vi "Test method finding benchmark.vi"() -> ()   [LabVIEW 2020]
uses:
  tests/Test Doubles/Test Case Test Double/Test Case Test Double.lvclass
  <vilib>/xml/Load XML File.vi
  <vilib>/xml/Close Reference(Node).vi
  <vilib>/xml/NI_XML.lvlib
  <resource>/objmgr/DOMUserDefRef.rc
  <vilib>/xml/Close Reference(NNMap).vi
panel:
  out "Array":path[](array[path])
  out "Array 7":path[](array[path])
  out "Numeric":i32
  out "Array 6":path[](array[path])
  out "appended array":path[](array[path])
  out "Array 2":path[](array[path])
  out "Array 5":path[](array[path])
  out "Array 4":string[](array[string])
  out "Array 3":path[](array[path])
  out "x-y":u32
  # "Name=\"_Test Dynamic Method.vi\" Type=\"VI\" URL=\"../_Test Dynamic Method.vi\">\n\t\t<Property Name=\"NI.ClassItem.ConnectorPane\" Type=\"Bin\">)!#!!!!!!!)!\"1!&amp;!!!-!%!!!@````]!!!!\"!!%!!!&amp;\"!!!!#1!-1#%'=X2B&gt;(6T!!!,1!-!\"'.P:'5!!\"\"!-0````]'=W^V=G.F!!!71&amp;!!!Q!!!!%!!AFF=H*P=C\"P&gt;81!\"!!!!%*!=!!?!!!@(62F=X1A1W&amp;T:3\"5:8.U)%2P&gt;7*M:3ZM&gt;G.M98.T!\"F5:8.U)%.B=W5A6'6T&gt;#\"%&lt;X6C&lt;'5A&lt;X6U!#\"!5!!$!!!!!1!#%W6S=G^S)'FO)#BO&lt;S\"F=H*P=CE!1E\"Q!\"Y!!\"]&gt;6'6T&gt;#\"$98.F)&amp;2F=X1A2'^V9GRF,GRW9WRB=X-!'&amp;2F=X1A1W&amp;T:3\"5:8.U)%2P&gt;7*M:3\"J&lt;A!!6!$Q!!Q!!Q!%!!1!\"1!%!!1!\"!!%!!9!\"!!%!!=$!!\"Y!!!.#!!!!!!!!!!!!!#.#Q!!!!!!!!!!!!!!!!!!!!!!!!I!!!!!!!!!!!!!!*)!!!!!!1!)!!!!!!</Property>\n\t\t<Property Name=\"NI.ClassItem.ExecutionSystem\" Type=\"Int\">-1</Property>\n\t\t<Property Name=\"NI.ClassItem.Flags\" Type=\"Int\">128</Property>\n\t\t<Property Name=\"NI.ClassItem.IsStaticMethod\" Type=\"Bool\">false</Property>\n\t\t<Property Name=\"NI.ClassItem.MethodScope\" Type=\"UInt\">1</Property>\n\t\t<Property Name=\"NI.ClassItem.Priority\" Type=\"Int\">1</Property>\n\t\t<Property Name=\"NI.ClassItem.State\" Type=\"Int\">1074541072</Property>"
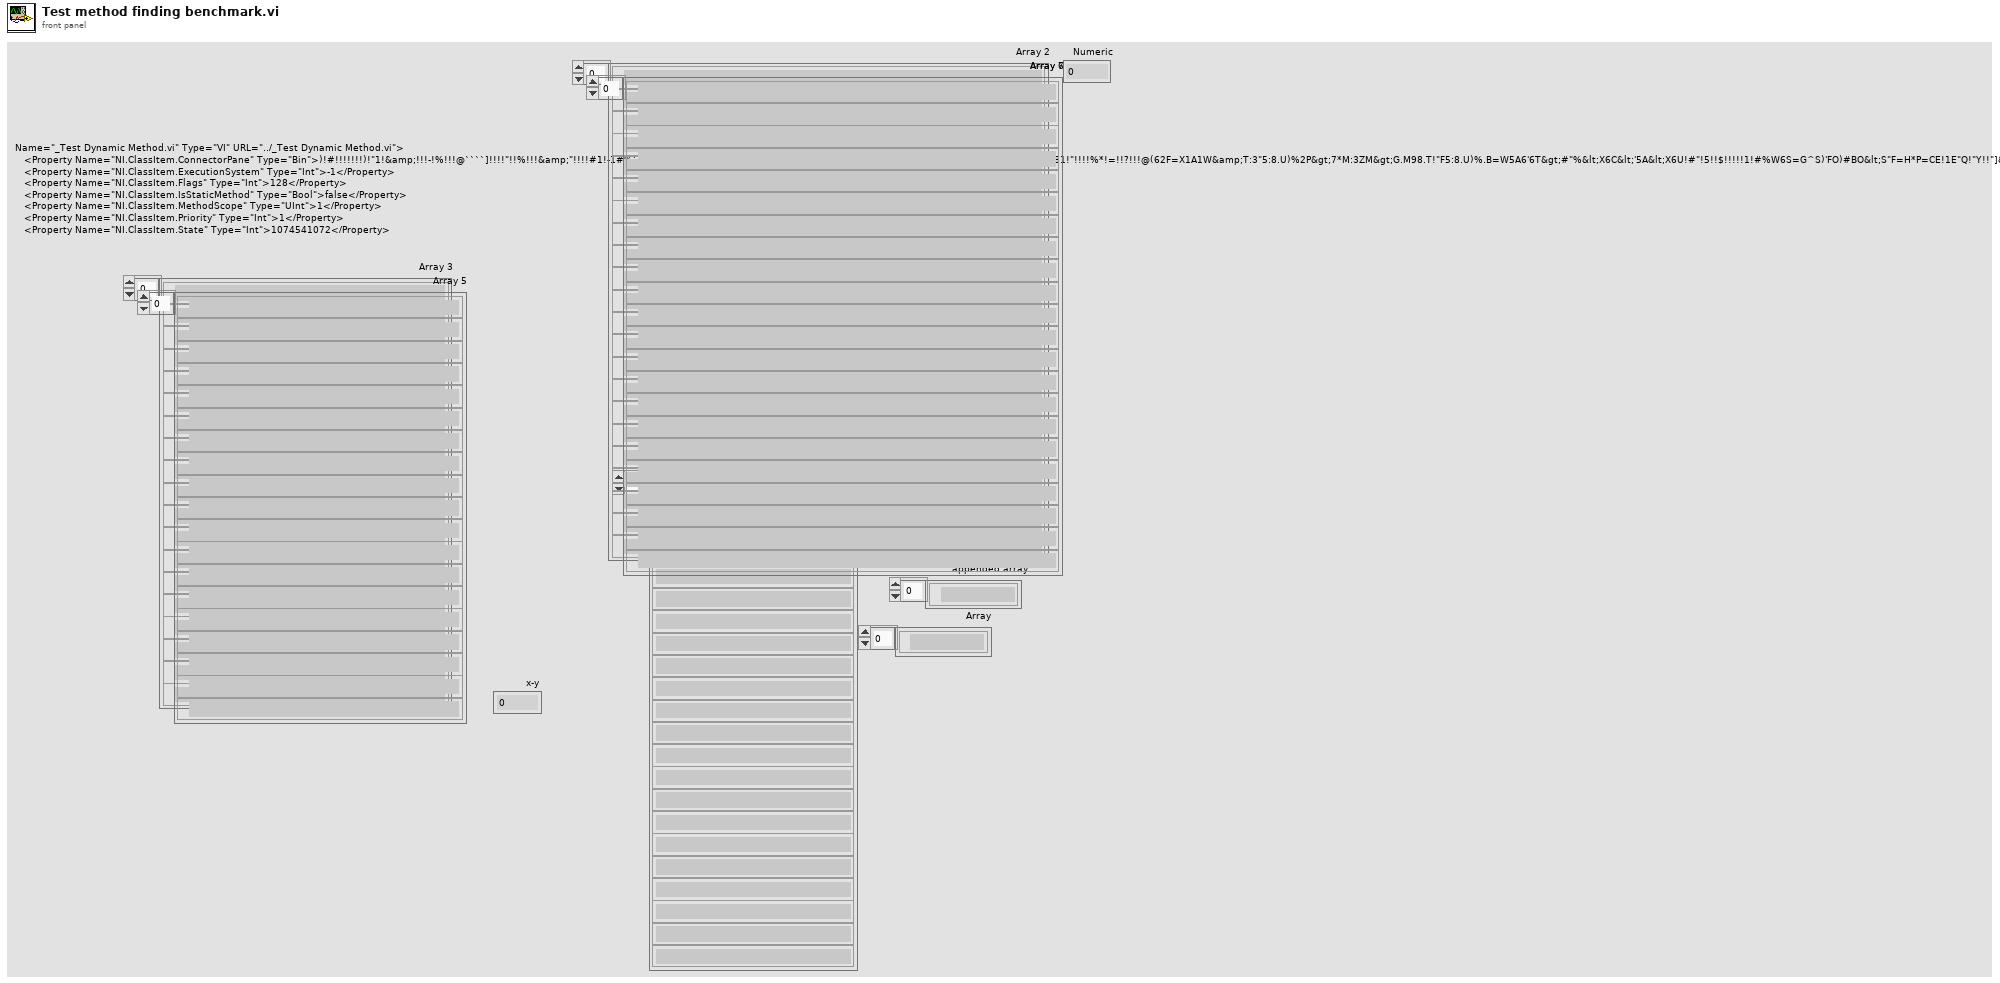
[diagram p1: front panel]
types:
  T1 = enum32{"invalid scope", "public", "private", "protected", "community"}
  T2 = enum16{"open", "replace", "create", "open or create", "replace or create", "replace or create with confirmation"}
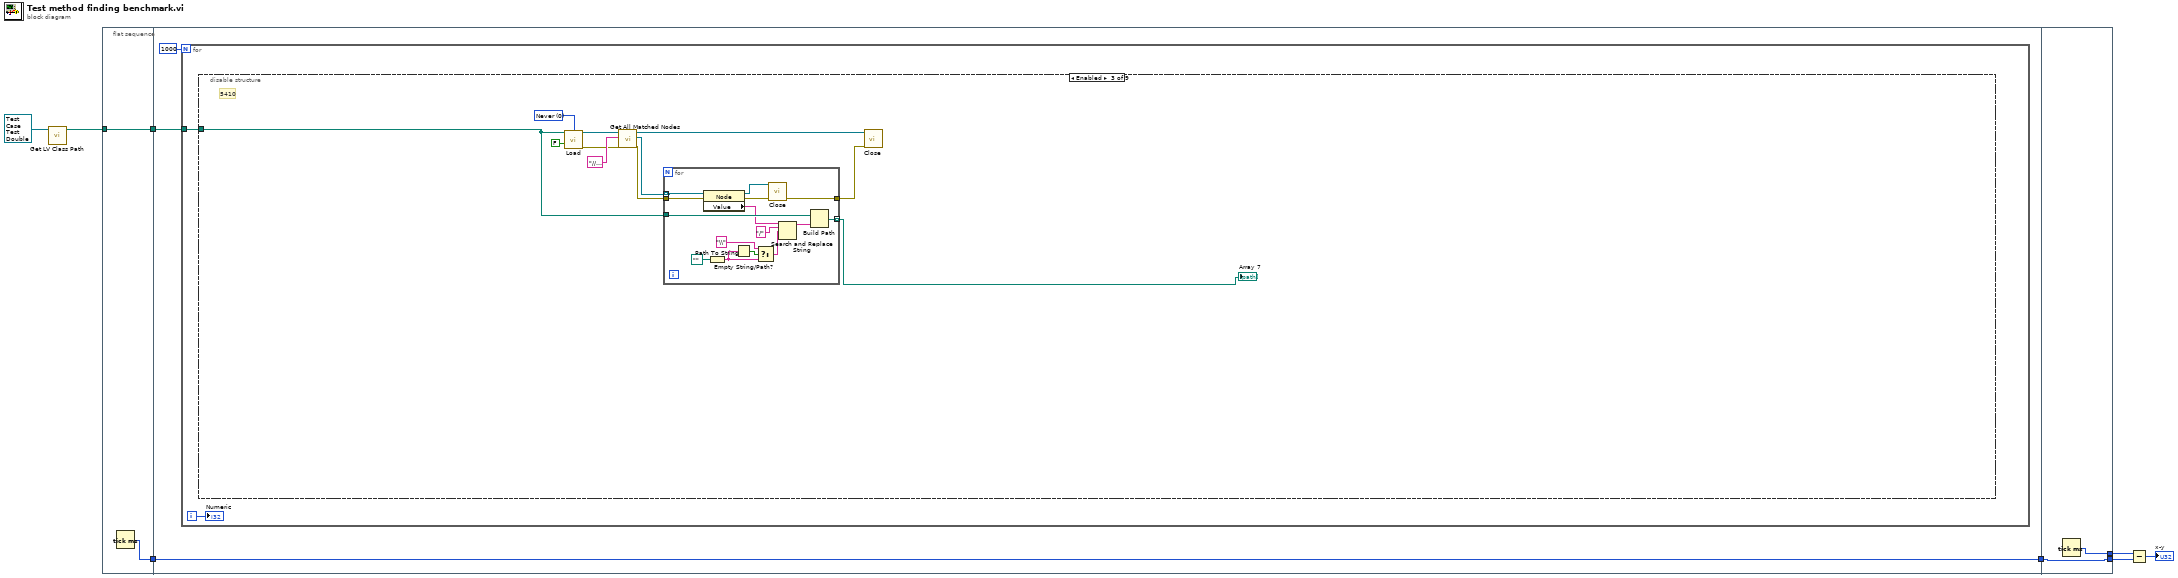
[diagram p0: block diagram]
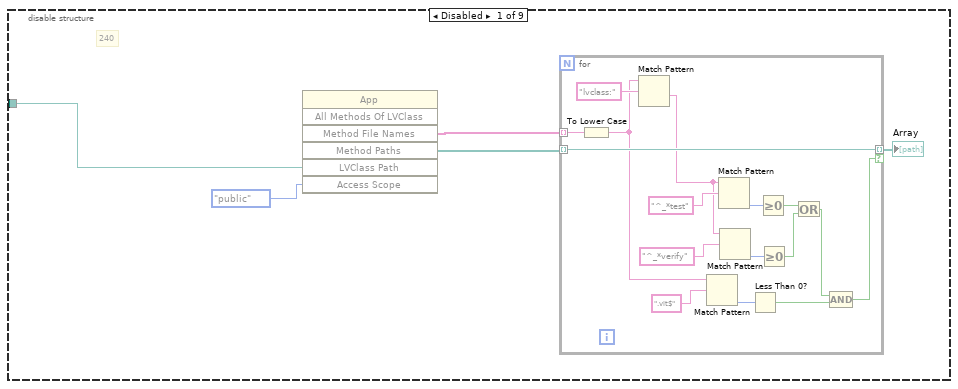
[diagram p2: hidden frame]
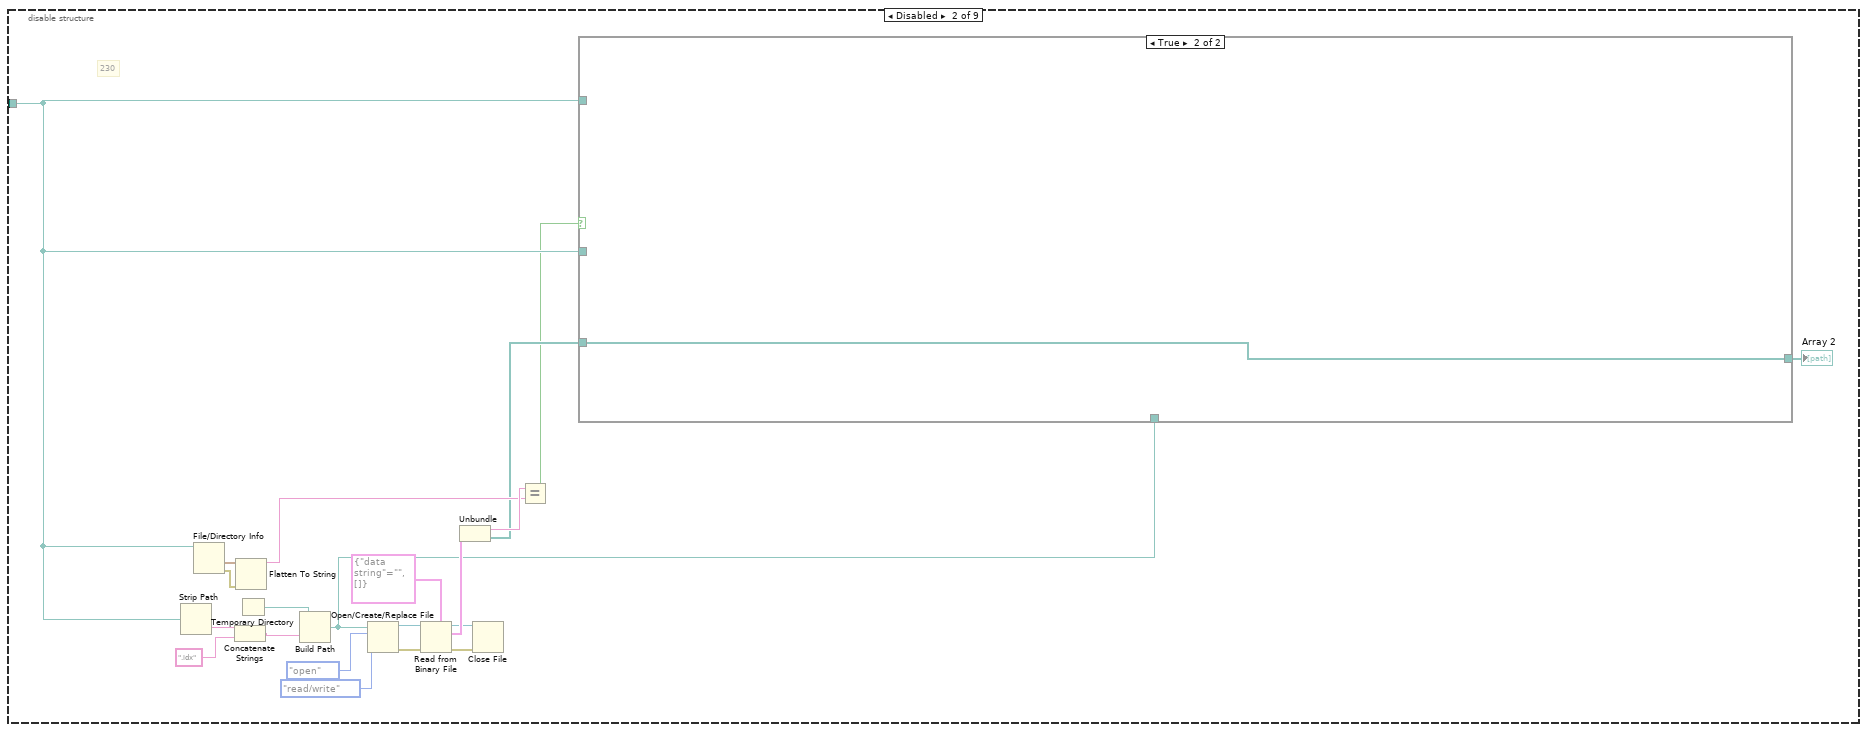
[diagram p3: hidden frame]
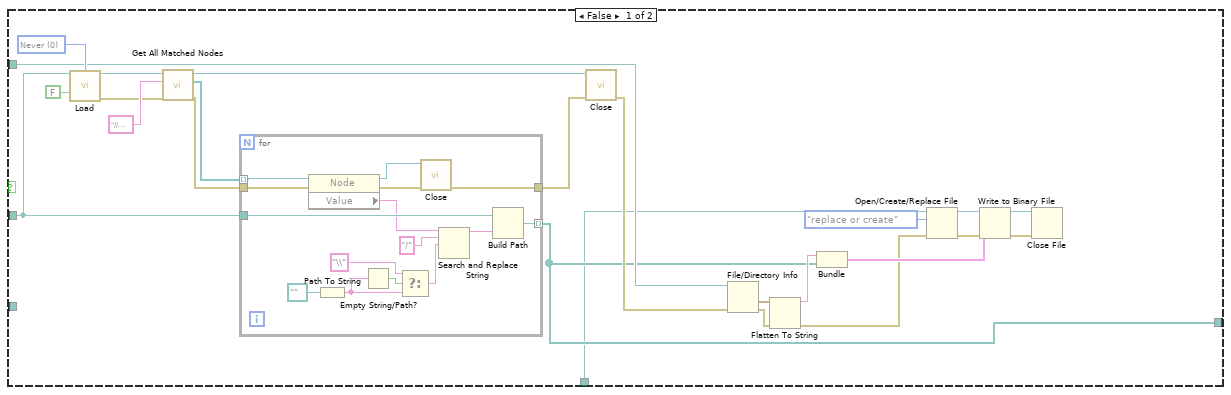
[diagram p4: hidden frame]
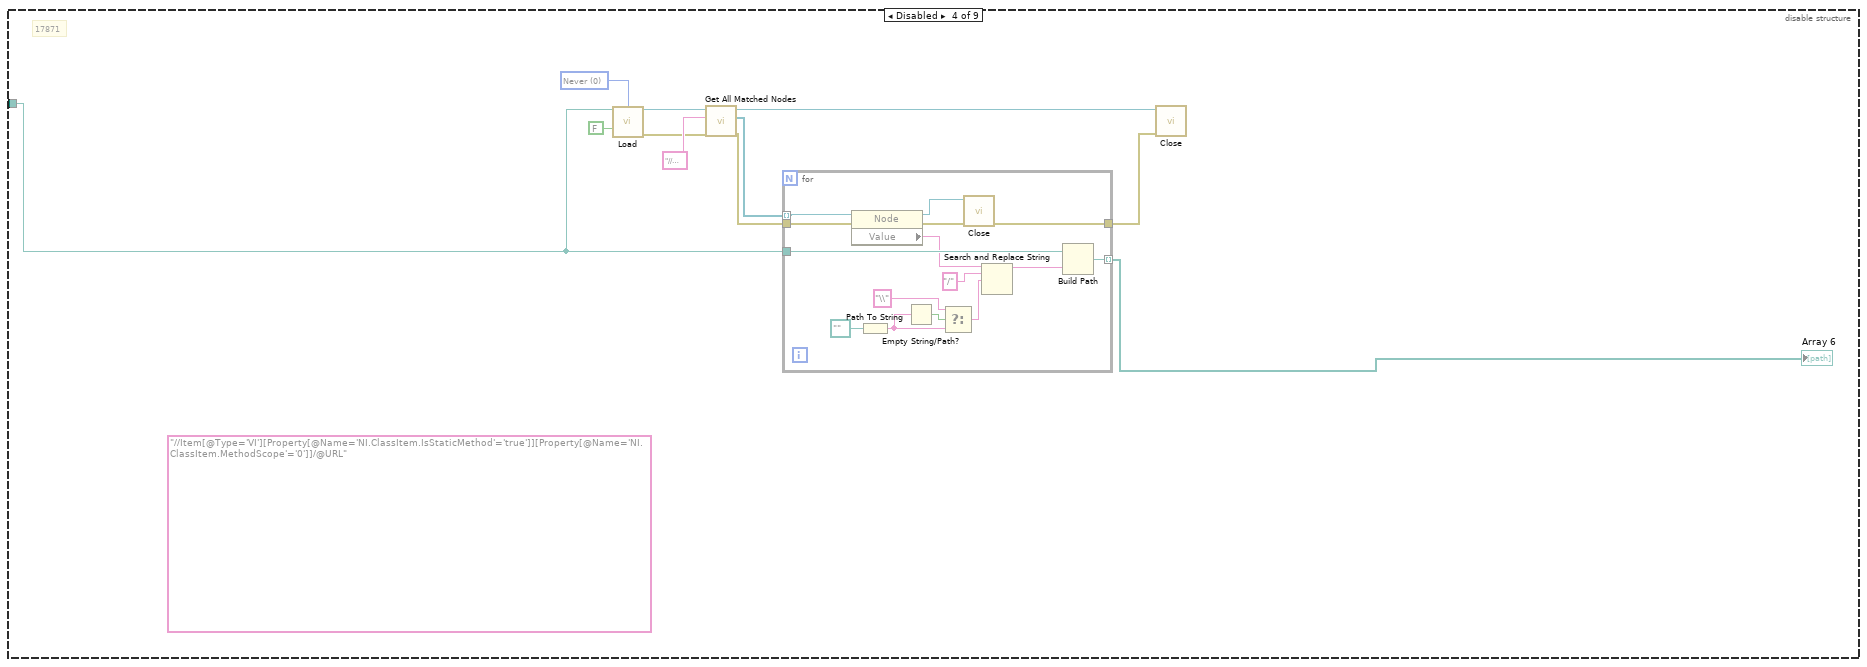
[diagram p5: hidden frame]
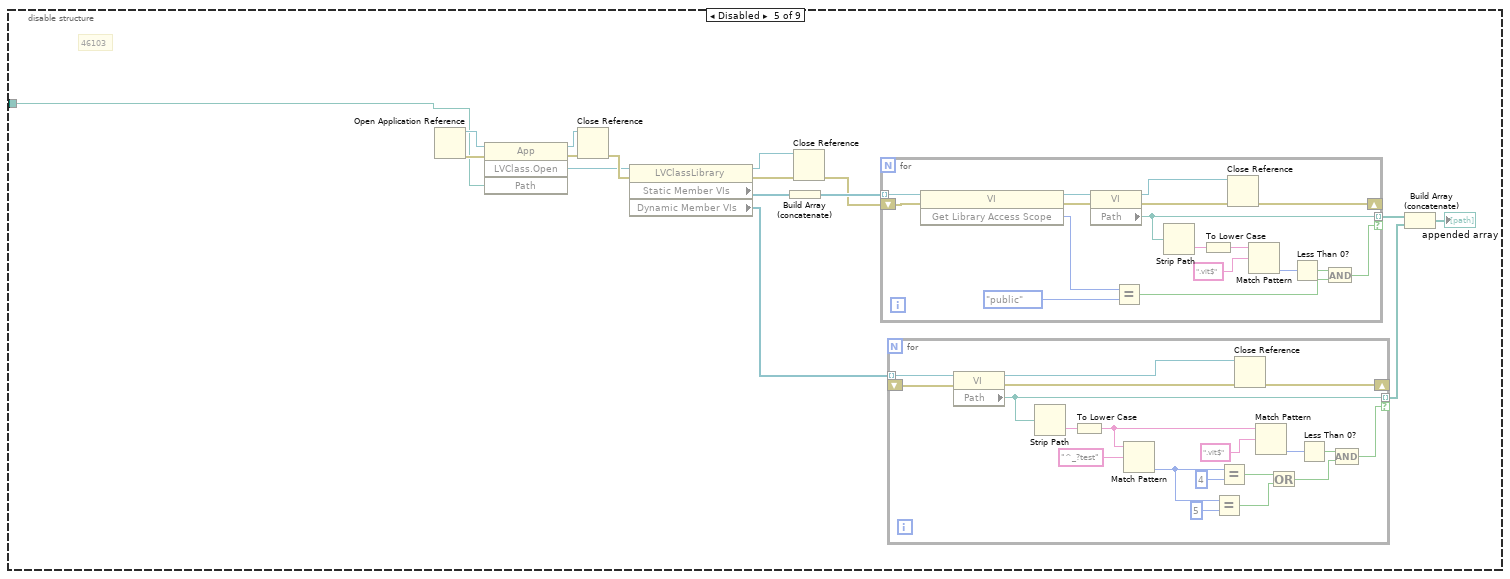
[diagram p6: hidden frame]
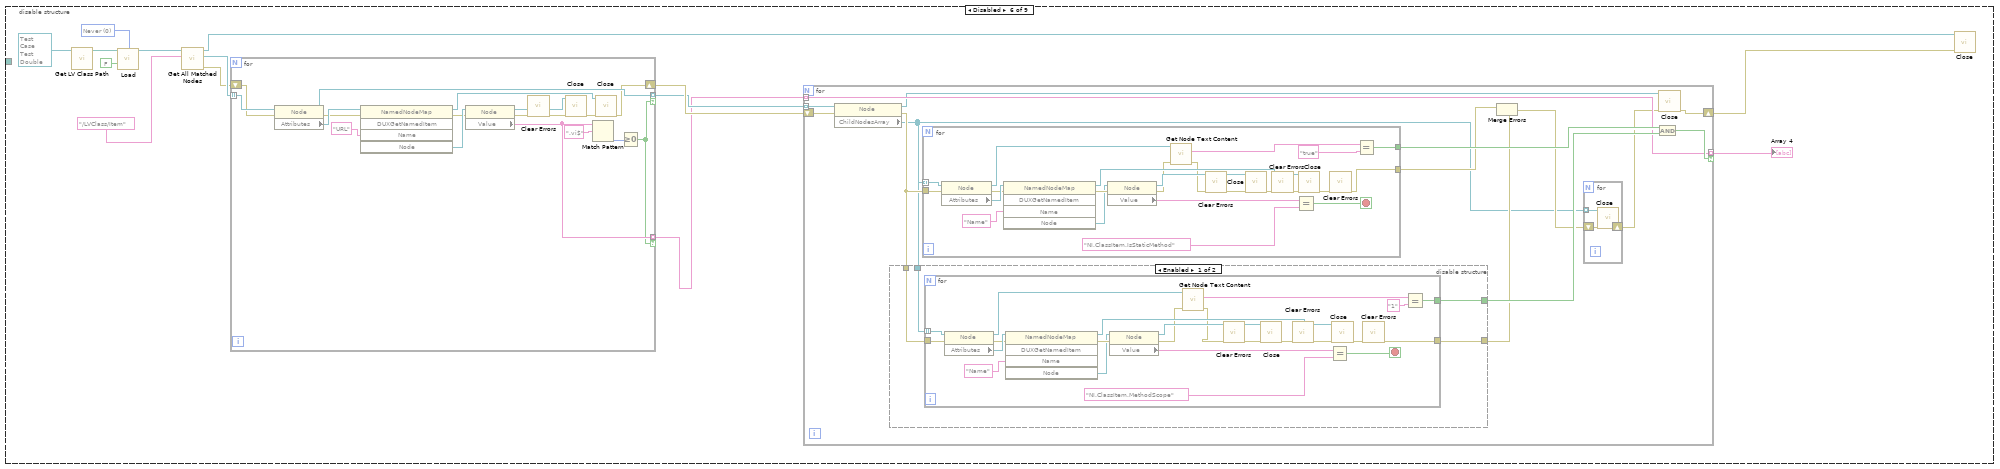
[diagram p7: hidden frame]
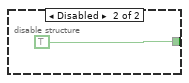
[diagram p8: hidden frame]
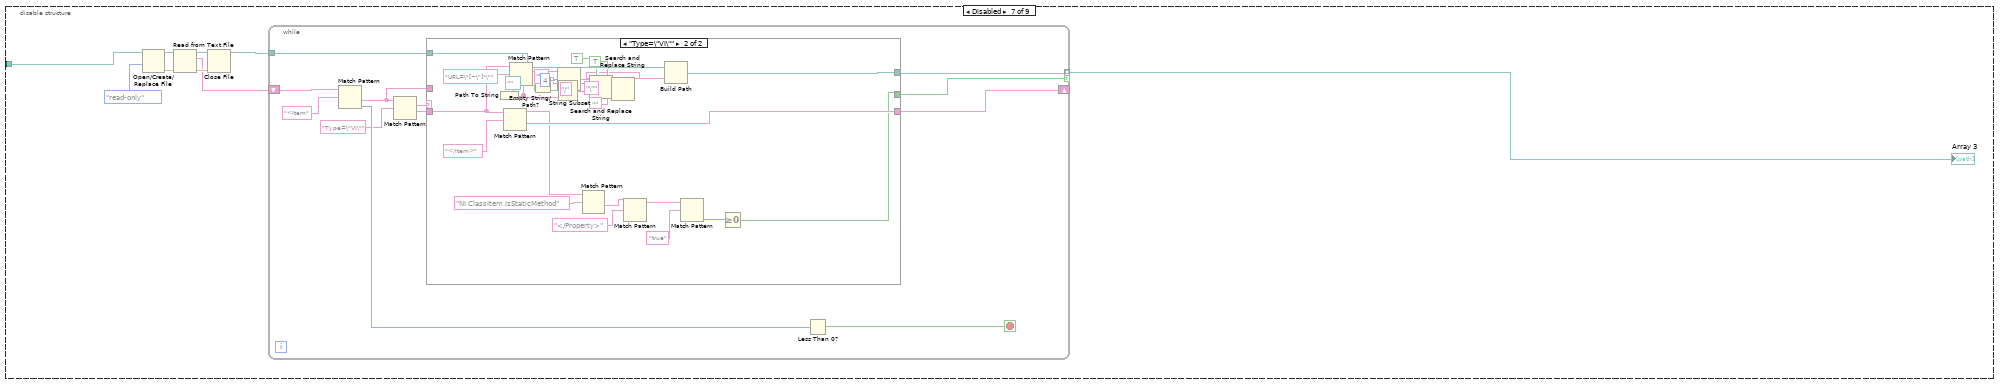
[diagram p9: hidden frame]
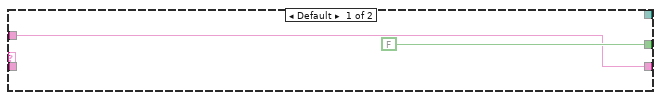
[diagram p10: hidden frame]
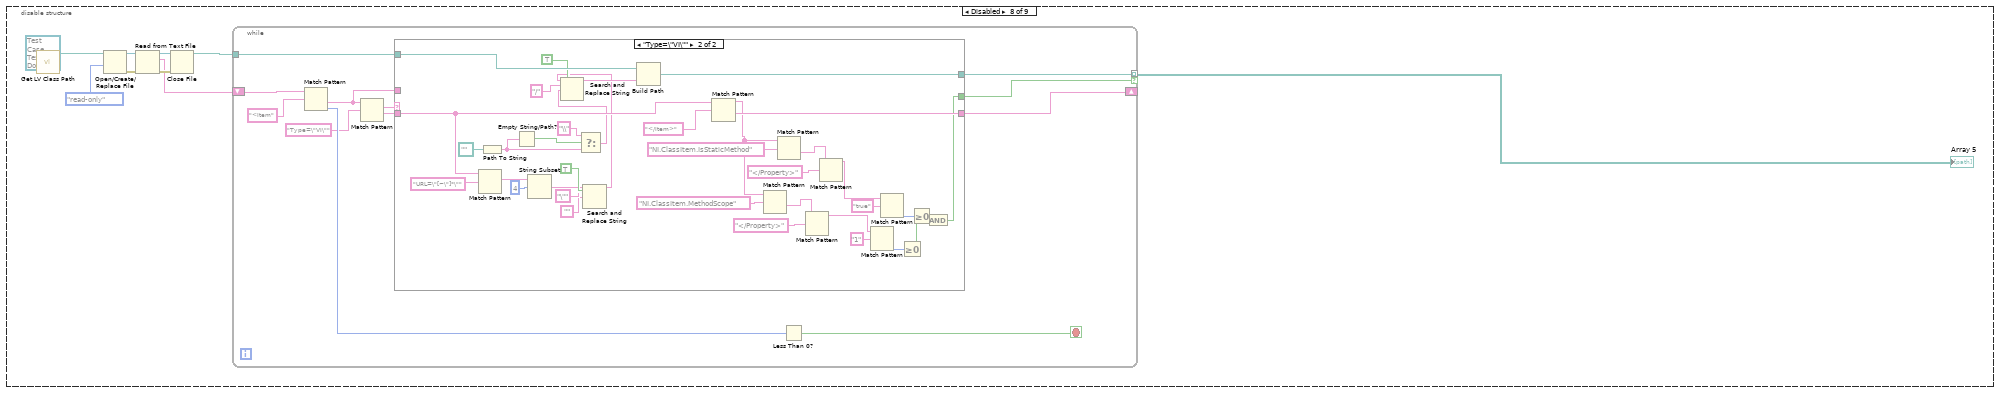
[diagram p11: hidden frame]
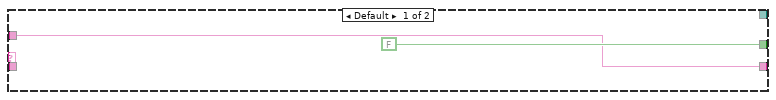
[diagram p12: hidden frame]
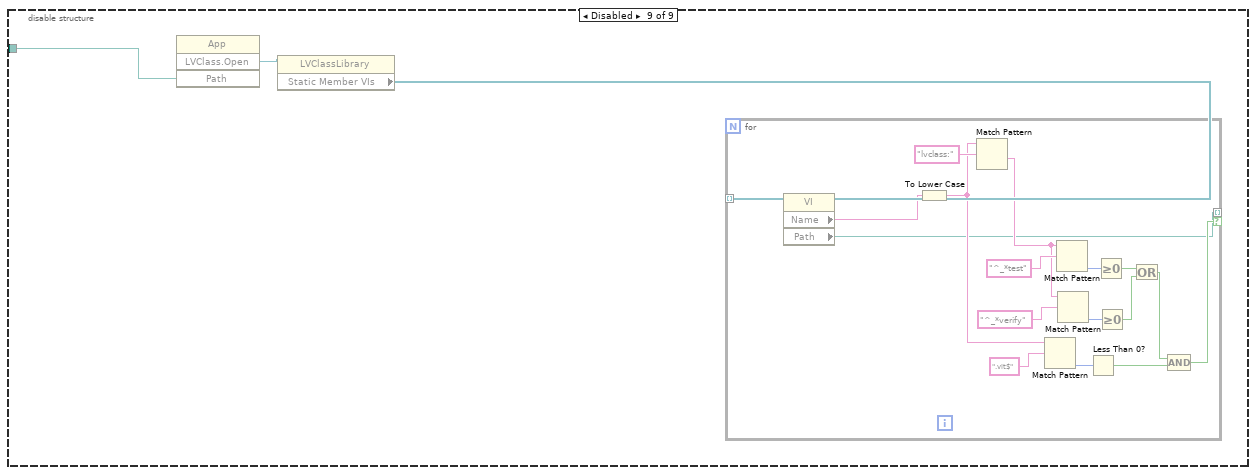
[diagram p13: hidden frame]
diagram:
  n1 = call <vilib>:"Get LV Class Path.vi"("object"=refnum<class "Test Case Test Double.lvclass"> refnum ("Test Case Test Double.lvclass")) -> ("class path"=w2:path)  [unwired: 9 in, 1 out]
  n2 = flat-sequence {
    tunnel: [w10] -> w7
    tunnel: [w9] -> w3
    tunnel: w2 -> [w9]
    tunnel: w7 -> [w13]
    tunnel: [w13] -> w6
    tunnel: w3 -> [w11]
    tunnel: [w437] -> w8
    tunnel: w6 -> [w436]
    tunnel: [w436] -> w5
    frame #0 {
      n3 = Tick Count (ms)() -> (millisecond timer value=w10:u32)
    }
    frame #1 {
      n4 = for {
        N: 1000 -> [_]
        tunnel: w11 -> [w15]
        i -> [w14]
        n5 = disable-structure shown="Enabled" {
          disable-tunnel: w15 -> [w16 w45 w107 w133 w151 _ w302 _ w415]
          frame Disabled {
            # "240"
            n6 = invoke class="App" method="All Methods Of LVClass"("LVClass Path"=w16, "Access Scope"=T1."public") -> ("Method File Names"=w18:string[], "Method Paths"=w19:path[])  [unwired: 5 in, 5 out]
            n7 = for {
              tunnel: [w32] -> w17 mode=indexing if=w33
              tunnel: w19 -> [w32] mode=indexing
              tunnel: w18 -> [w28] mode=indexing
              n8 = To Lower Case(string=w28) -> (all lower case string=w22:string)
              n9 = Match Pattern(string=w22, regular expression="lvclass:") -> (after substring=w29:string)  [unwired: 1 in, 3 out]
              n10 = Match Pattern(string=w22, regular expression=".vit$") -> (offset past match=w35:i32)  [unwired: 1 in, 3 out]
              n11 = Match Pattern(string=w29, regular expression="^_*test") -> (offset past match=w31:i32)  [unwired: 1 in, 3 out]
              n12 = Match Pattern(string=w29, regular expression="^_*verify") -> (offset past match=w25:i32)  [unwired: 1 in, 3 out]
              n13 = Less Than 0?(x=w35) -> (x < 0?=w34:bool)
              n14 = Greater Or Equal To 0?(x=w31) -> (x >= 0?=w23:bool)
              n15 = Greater Or Equal To 0?(x=w25) -> (x >= 0?=w24:bool)
              n16 = Or(x=w23, y=w24) -> (x .or. y?=w21:bool)
              n17 = Compound Arithmetic op=AND(w21, w34) -> (w33:bool)
            }
            "Array" <- w17
          }
          frame Disabled {
            # "230"
            n18 = Strip Path(path=w45) -> (name=w57:string)  [unwired: 1 out]
            n19 = File/Directory Info(path=w45) -> (last mod=w43:timestamp, error out=w44:errorcluster)  [unwired: 1 in, 5 out]
            n20 = Concatenate Strings(w57, ".idx" ("string")) -> (w54:string)
            n21 = Flatten To String(anything=w43, error in (no error)=w44) -> (data string=w49:string)  [unwired: 2 in, 2 out]
            n22 = Temporary Directory() -> (w55:path)
            n23 = Build Path(base path=w55, name or relative path=w54) -> (appended path=w47:path)
            n24 = Open/Create/Replace File(file path (use dialog)=w47, operation (0:open)=T2."open", access (0:read/write)=enum16{"read/write", "read-only", "write-only"}."read/write") -> (refnum out=w42:refnum<file>, error out=w41:errorcluster)  [unwired: 3 in, 1 out]
            n25 = Read from Binary File(5:cluster{"data string":string, path[]} {"data string"="", []} ("output cluster"), 8:w41, 11:w42) -> (0:w39:errorcluster, 2:w51:cluster{"data string":string, path[]}, 3:w40:refnum<file>)  [unwired: 3 in, 1 out]
            n26 = Unbundle(w51) -> ("data string"=w50:string, w48:path[])
            n27 = Close File(refnum=w40, error in=w39) -> ()  [unwired: 2 out]
            n28 = Equal?(x=w50, y=w49) -> (x = y?=w37:bool)
            n29 = case shown="True" w37 {
              tunnel: [w66 w97] -> w46
              tunnel: w45 -> [w72 _]
              tunnel: w48 -> [_ w97]
              tunnel: w45 -> [w68 _]
              tunnel: w47 -> [w61 _]
              frame False {
                w81 = 0 items=["Never", "Always", "Auto"] ("validate on load (Auto)")
                n30 = call-poly <vilib>:"Load.vi"("path to XML document"=w72, "validate on load (Auto)"=w81, "load external DTD (True)"=FALSE) -> ("DOM document out"=w79:refnum<k20>, "error out"=w73:errorcluster)  [unwired: 10 in, 1 out]
                n31 = call <vilib>:"Get All Matched Nodes.vi"("error in (no error)"=w73, "XPath expression"="//Item[@Type='VI'][Property[@Name='NI.ClassItem.IsStaticMethod'='true']][Property[@Name='NI.ClassItem.MethodScope'='0']]/@URL", "node in"=w79) -> ("error out"=w75:errorcluster, "node result array"=w77:refnum<k20>[], "node out"=w76:refnum<k20>)  [unwired: 6 out]
                n32 = for {
                  tunnel: w77 -> [w96] mode=indexing
                  tunnel: w75 -> [w95]
                  tunnel: [w92] -> w74
                  tunnel: w72 -> [w84]
                  tunnel: [w83] -> w66 mode=indexing
                  n33 = property class="Node"(reference=w96, error in=w95) -> (reference out=w94:refnum<k20>, error out=w93:errorcluster, "Value"=w82:string)
                  n34 = Path To String(path=path "") -> (string=w90:string)
                  n35 = Empty String/Path?(string/path=w90) -> (empty?=w89:bool)
                  n36 = Select(t="\\" ("search string"), s=w89, f=w90) -> (s? t:f=w88:string)
                  n37 = call-poly <vilib>:"Close.vi"("error in (no error)"=w93, "node"=w94) -> ("error out"=w92:errorcluster)  [unwired: 7 out]
                  n38 = Search and Replace String(input string=w82, search string="/", replace string=w88) -> (result string=w91:string)  [unwired: 5 in, 3 out]
                  n39 = Build Path(base path=w84, name or relative path=w91) -> (appended path=w83:path)
                }
                n40 = call-poly <vilib>:"Close.vi"("error in (no error)"=w74, "node"=w76) -> ("error out"=w69:errorcluster)  [unwired: 7 out]
                n41 = File/Directory Info(path=w68, error in=w69) -> (last mod=w70:timestamp, error out=w71:errorcluster)  [unwired: 5 out]
                n42 = Flatten To String(anything=w70, error in (no error)=w71) -> (data string=w67:string, error out=w58:errorcluster)  [unwired: 2 in, 1 out]
                n43 = Bundle("data string"=w67, w66) -> (w60:cluster{"data string":string, path[]})  [unwired: 1 in]
                n44 = Open/Create/Replace File(file path (use dialog)=w61, error in=w58, operation (0:open)=T2."replace or create") -> (refnum out=w62:refnum<file>, error out=w63:errorcluster)  [unwired: 3 in, 1 out]
                n45 = Write to Binary File(file (use dialog)=w62, data=w60, error in=w63) -> (refnum out=w64:refnum<file>, error out=w65:errorcluster)  [unwired: 3 in, 1 out]
                n46 = Close File(refnum=w64, error in=w65) -> ()  [unwired: 2 out]
              }
              frame True {
              }
            }
            "Array 2" <- w46
          }
          frame Enabled {
            w106 = 0 items=["Never", "Always", "Auto"] ("validate on load (Auto)")
            # "5410"
            n47 = call-poly <vilib>:"Load.vi"("path to XML document"=w107, "validate on load (Auto)"=w106, "load external DTD (True)"=FALSE) -> ("DOM document out"=w104:refnum<k20>, "error out"=w98:errorcluster)  [unwired: 10 in, 1 out]
            n48 = call <vilib>:"Get All Matched Nodes.vi"("error in (no error)"=w98, "XPath expression"="//Item[@Type='VI'][Property[@Name='NI.ClassItem.IsStaticMethod'='true']][Property[@Name='NI.ClassItem.MethodScope'='0']]/@URL", "node in"=w104) -> ("error out"=w100:errorcluster, "node result array"=w102:refnum<k20>[], "node out"=w101:refnum<k20>)  [unwired: 6 out]
            n49 = for {
              tunnel: w102 -> [w123] mode=indexing
              tunnel: w100 -> [w122]
              tunnel: [w119] -> w99
              tunnel: w107 -> [w111]
              tunnel: [w110] -> w108 mode=indexing
              n50 = property class="Node"(reference=w123, error in=w122) -> (reference out=w121:refnum<k20>, error out=w120:errorcluster, "Value"=w109:string)
              n51 = Path To String(path=path "") -> (string=w117:string)
              n52 = Empty String/Path?(string/path=w117) -> (empty?=w116:bool)
              n53 = Select(t="\\" ("search string"), s=w116, f=w117) -> (s? t:f=w115:string)
              n54 = call-poly <vilib>:"Close.vi"("error in (no error)"=w120, "node"=w121) -> ("error out"=w119:errorcluster)  [unwired: 7 out]
              n55 = Search and Replace String(input string=w109, search string="/", replace string=w115) -> (result string=w118:string)  [unwired: 5 in, 3 out]
              n56 = Build Path(base path=w111, name or relative path=w118) -> (appended path=w110:path)
            }
            "Array 7" <- w108
            n57 = call-poly <vilib>:"Close.vi"("error in (no error)"=w99, "node"=w101) -> ()  [unwired: 8 out]
          }
          frame Disabled {
            (unwired) "//Item[@Type='VI'][Property[@Name='NI.ClassItem.IsStaticMethod'='true']][Property[@Name='NI.ClassItem.MethodScope'='0']]/@URL" ("XPath expression")
            w132 = 0 items=["Never", "Always", "Auto"] ("validate on load (Auto)")
            # "17871"
            n58 = call-poly <vilib>:"Load.vi"("path to XML document"=w133, "validate on load (Auto)"=w132, "load external DTD (True)"=FALSE) -> ("DOM document out"=w130:refnum<k20>, "error out"=w124:errorcluster)  [unwired: 10 in, 1 out]
            n59 = call <vilib>:"Get All Matched Nodes.vi"("error in (no error)"=w124, "XPath expression"="//Item[@Type='VI'][Property[@Name='NI.ClassItem.IsStaticMethod']='true'][Property[@Name='NI.ClassItem.MethodScope']='1']/@URL", "node in"=w130) -> ("error out"=w126:errorcluster, "node result array"=w128:refnum<k20>[], "node out"=w127:refnum<k20>)  [unwired: 6 out]
            n60 = for {
              tunnel: w128 -> [w149] mode=indexing
              tunnel: w126 -> [w148]
              tunnel: [w145] -> w125
              tunnel: w133 -> [w137]
              tunnel: [w136] -> w134 mode=indexing
              n61 = property class="Node"(reference=w149, error in=w148) -> (reference out=w147:refnum<k20>, error out=w146:errorcluster, "Value"=w135:string)
              n62 = Path To String(path=path "") -> (string=w143:string)
              n63 = Empty String/Path?(string/path=w143) -> (empty?=w142:bool)
              n64 = Select(t="\\" ("search string"), s=w142, f=w143) -> (s? t:f=w141:string)
              n65 = call-poly <vilib>:"Close.vi"("error in (no error)"=w146, "node"=w147) -> ("error out"=w145:errorcluster)  [unwired: 7 out]
              n66 = Search and Replace String(input string=w135, search string="/", replace string=w141) -> (result string=w144:string)  [unwired: 5 in, 3 out]
              n67 = Build Path(base path=w137, name or relative path=w144) -> (appended path=w136:path)
            }
            "Array 6" <- w134
            n68 = call-poly <vilib>:"Close.vi"("error in (no error)"=w125, "node"=w127) -> ()  [unwired: 8 out]
          }
          frame Disabled {
            # "46103"
            n69 = Open Application Reference() -> (0:w164:errorcluster, 3:w165:refnum<vi>)  [unwired: 4 in]
            n70 = invoke class="App" method="LVClass.Open"(reference=w165, error in=w164, "Path"=w151) -> (reference out=w159:refnum<vi>, error out=w163:errorcluster, "LVClass.Open"=w157:refnum<vi>)  [unwired: 1 in, 1 out]
            n71 = Close Reference(reference=w159, error in (no error)=w163) -> (error out=w160:errorcluster)
            n72 = property class="LVClassLibrary"(reference=w157, error in=w160) -> (reference out=w154:refnum<vi>, error out=w156:errorcluster, "Static Member VIs"=w162:refnum<vi>[], "Dynamic Member VIs"=w153:refnum<vi>[])
            n73 = Build Array (concatenate)(w162) -> (w158:refnum<vi>[])
            n74 = Close Reference(reference=w154, error in (no error)=w156) -> (error out=w155:errorcluster)
            n75 = for {
              tunnel: w158 -> [w171] mode=indexing
              tunnel: [w179] -> w161 mode=indexing if=w167
              shift-right: [w180] -> _
              shift-left: w155 -> [w182]
              n76 = invoke class="VI" method="Get Library Access Scope"(reference=w171, error in=w182) -> (reference out=w170:refnum<vi>, error out=w172:errorcluster, "Get Library Access Scope"=w169:T1)  [unwired: 1 in]
              n77 = property class="VI"(reference=w170, error in=w172) -> (reference out=w173:refnum<vi>, error out=w181:errorcluster, "Path"=w179:path)
              n78 = Equal?(x=w169, y=T1."public") -> (x = y?=w166:bool)
              n79 = Strip Path(path=w179) -> (name=w178:string)  [unwired: 1 out]
              n80 = To Lower Case(string=w178) -> (all lower case string=w174:string)
              n81 = Close Reference(reference=w173, error in (no error)=w181) -> (error out=w180:errorcluster)
              n82 = Match Pattern(string=w174, regular expression=".vit$") -> (offset past match=w176:i32)  [unwired: 1 in, 3 out]
              n83 = Less Than 0?(x=w176) -> (x < 0?=w175:bool)
              n84 = And(x=w175, y=w166) -> (x .and. y?=w167:bool)
            }
            n85 = for {
              tunnel: w153 -> [w192] mode=indexing
              tunnel: [w199] -> w152 mode=indexing if=w191
              shift-right: [w200] -> _
              shift-left: _ -> [w193]
              n86 = property class="VI"(reference=w192, error in=w193) -> (reference out=w194:refnum<vi>, error out=w201:errorcluster, "Path"=w199:path)
              n87 = Strip Path(path=w199) -> (name=w198:string)  [unwired: 1 out]
              n88 = To Lower Case(string=w198) -> (all lower case string=w189:string)
              n89 = Match Pattern(string=w189, regular expression="^_?test" ("string")) -> (offset past match=w184:i32)  [unwired: 1 in, 3 out]
              n90 = Equal?(x=w184, y=5) -> (x = y?=w183:bool)
              n91 = Equal?(x=w184, y=4) -> (x = y?=w187:bool)
              n92 = Close Reference(reference=w194, error in (no error)=w201) -> (error out=w200:errorcluster)
              n93 = Match Pattern(string=w189, regular expression=".vit$") -> (offset past match=w196:i32)  [unwired: 1 in, 3 out]
              n94 = Or(x=w187, y=w183) -> (x .or. y?=w186:bool)
              n95 = Less Than 0?(x=w196) -> (x < 0?=w195:bool)
              n96 = Compound Arithmetic op=AND(w195, w186) -> (w191:bool)
            }
            n97 = Build Array (concatenate)(w161, w152) -> (→"appended array":path[])
          }
          frame Disabled {
            w213 = 0 items=["Never", "Always", "Auto"] ("validate on load (Auto)")
            n98 = call <vilib>:"Get LV Class Path.vi"("object"=refnum<class "Test Case Test Double.lvclass"> refnum ("Test Case Test Double.lvclass")) -> ("class path"=w214:path)  [unwired: 9 in, 1 out]
            n99 = call-poly <vilib>:"Load.vi"("path to XML document"=w214, "validate on load (Auto)"=w213, "load external DTD (True)"=FALSE) -> ("DOM document out"=w211:refnum<k20>)  [unwired: 10 in, 2 out]
            n100 = call <vilib>:"Get All Matched Nodes.vi"("XPath expression"="/LVClass/Item", "node in"=w211) -> ("error out"=w207:errorcluster, "node result array"=w209:refnum<k20>[], "node out"=w208:refnum<k20>)  [unwired: 1 in, 6 out]
            n101 = for {
              tunnel: w209 -> [w301] mode=indexing
              shift-right: [w286] -> w206
              shift-left: w207 -> [w291]
              tunnel: [w300] -> w204 mode=indexing if=w284
              tunnel: [w296] -> w203 mode=indexing if=w284
              n102 = property class="Node"(reference=w301, error in=w291) -> (reference out=w300:refnum<k20>, error out=w292:errorcluster, "Attributes"=w297:refnum<k20>)
              n103 = invoke on="Invoke Node" class="NamedNodeMap" method="DUXGetNamedItem"(reference=w297, error in=w292, "Name"="URL") -> (reference out=w293:refnum<k20>, error out=w288:errorcluster, "Node"=w299:refnum<k20>)  [unwired: 2 in, 2 out]
              n104 = property class="Node"(reference=w299, error in=w288) -> (reference out=w290:refnum<k20>, error out=w289:errorcluster, "Value"=w296:string)
              n105 = call <vilib>:"Clear Errors.vi"("error in (no error)"=w289) -> ("error out"=w285:errorcluster)  [unwired: 5 in, 1 out]
              n106 = call-poly <vilib>:"Close.vi"("error in (no error)"=w285, "node"=w290) -> ("error out"=w287:errorcluster)  [unwired: 7 in]
              n107 = Match Pattern(string=w296, regular expression=".vi$") -> (offset past match=w294:i32)  [unwired: 1 in, 3 out]
              n108 = call-poly <vilib>:"Close.vi"("error in (no error)"=w287, "named node map"=w293) -> ("error out"=w286:errorcluster)  [unwired: 7 in]
              n109 = Greater Or Equal To 0?(x=w294) -> (x >= 0?=w284:bool)
            }
            n110 = for {
              shift-right: [w219] -> w205
              shift-left: w206 -> [w229]
              tunnel: w204 -> [w228] mode=indexing
              tunnel: [w224] -> w202 mode=indexing if=w226
              tunnel: w203 -> [w224] mode=indexing
              n111 = property class="Node"(reference=w228, error in=w229) -> (reference out=w223:refnum<k20>, error out=w222:errorcluster, "ChildNodesArray"=w216:refnum<k20>[])
              n112 = disable-structure shown="Enabled" {
                disable-tunnel: w216 -> [w236 _]
                disable-tunnel: [w235 TRUE] -> w225
                disable-tunnel: w222 -> [w234 _]
                disable-tunnel: [w233 _] -> w221
                frame Enabled {
                  n113 = for {
                    tunnel: w236 -> [w259] mode=indexing
                    tunnel: [w248] -> w235
                    tunnel: w234 -> [w245]
                    tunnel: [w241] -> w233
                    stop <- w253 stop-if-true
                    n114 = property class="Node"(reference=w259, error in=w245) -> (reference out=w251:refnum<k20>, error out=w244:errorcluster, "Attributes"=w257:refnum<k20>)
                    n115 = invoke on="Invoke Node" class="NamedNodeMap" method="DUXGetNamedItem"(reference=w257, error in=w244, "Name"="Name") -> (reference out=w247:refnum<k20>, error out=w256:errorcluster, "Node"=w252:refnum<k20>)  [unwired: 2 in, 2 out]
                    n116 = property class="Node"(reference=w252, error in=w256) -> (reference out=w246:refnum<k20>, error out=w239:errorcluster, "Value"=w254:string)
                    n117 = call <vilib>:"Get Node Text Content.vi"("error in (no error)"=w239, "node in"=w251) -> ("error out"=w238:errorcluster, "node text"=w250:string)  [unwired: 7 in, 1 out]
                    n118 = call <vilib>:"Clear Errors.vi"("error in (no error)"=w238) -> ("error out"=w240:errorcluster)  [unwired: 5 in, 1 out]
                    n119 = call-poly <vilib>:"Close.vi"("error in (no error)"=w240, "node"=w246) -> ("error out"=w243:errorcluster)  [unwired: 7 in]
                    n120 = call <vilib>:"Clear Errors.vi"("error in (no error)"=w243) -> ("error out"=w237:errorcluster)  [unwired: 5 in, 1 out]
                    n121 = Equal?(x=w254, y="NI.ClassItem.MethodScope" ("Name")) -> (x = y?=w253:bool)
                    n122 = call-poly <vilib>:"Close.vi"("error in (no error)"=w237, "named node map"=w247) -> ("error out"=w242:errorcluster)  [unwired: 7 in]
                    n123 = call <vilib>:"Clear Errors.vi"("error in (no error)"=w242) -> ("error out"=w241:errorcluster)  [unwired: 5 in, 1 out]
                    n124 = Equal?(x=w250, y="1") -> (x = y?=w248:bool)
                  }
                }
                frame Disabled {
                }
              }
              n125 = for {
                tunnel: w216 -> [w283] mode=indexing
                tunnel: [w272] -> w227
                tunnel: w222 -> [w269]
                tunnel: [w261] -> w220
                stop <- w277 stop-if-true
                n126 = property class="Node"(reference=w283, error in=w269) -> (reference out=w275:refnum<k20>, error out=w268:errorcluster, "Attributes"=w281:refnum<k20>)
                n127 = invoke on="Invoke Node" class="NamedNodeMap" method="DUXGetNamedItem"(reference=w281, error in=w268, "Name"="Name") -> (reference out=w271:refnum<k20>, error out=w280:errorcluster, "Node"=w276:refnum<k20>)  [unwired: 2 in, 2 out]
                n128 = property class="Node"(reference=w276, error in=w280) -> (reference out=w270:refnum<k20>, error out=w264:errorcluster, "Value"=w278:string)
                n129 = call <vilib>:"Get Node Text Content.vi"("error in (no error)"=w264, "node in"=w275) -> ("error out"=w263:errorcluster, "node text"=w274:string)  [unwired: 7 in, 1 out]
                n130 = call <vilib>:"Clear Errors.vi"("error in (no error)"=w263) -> ("error out"=w265:errorcluster)  [unwired: 5 in, 1 out]
                n131 = call-poly <vilib>:"Close.vi"("error in (no error)"=w265, "node"=w270) -> ("error out"=w267:errorcluster)  [unwired: 7 in]
                n132 = call <vilib>:"Clear Errors.vi"("error in (no error)"=w267) -> ("error out"=w262:errorcluster)  [unwired: 5 in, 1 out]
                n133 = Equal?(x=w278, y="NI.ClassItem.IsStaticMethod" ("Name")) -> (x = y?=w277:bool)
                n134 = call-poly <vilib>:"Close.vi"("error in (no error)"=w262, "named node map"=w271) -> ("error out"=w266:errorcluster)  [unwired: 7 in]
                n135 = call <vilib>:"Clear Errors.vi"("error in (no error)"=w266) -> ("error out"=w261:errorcluster)  [unwired: 5 in, 1 out]
                n136 = Equal?(x=w274, y="true") -> (x = y?=w272:bool)
              }
              n137 = Merge Errors(w220, w221) -> (w218:errorcluster)
              n138 = for {
                shift-right: [w231] -> w217
                shift-left: w218 -> [w232]
                tunnel: w216 -> [w230] mode=indexing
                n139 = call-poly <vilib>:"Close.vi"("error in (no error)"=w232, "node"=w230) -> ("error out"=w231:errorcluster)  [unwired: 7 in]
              }
              n140 = And(x=w227, y=w225) -> (x .and. y?=w226:bool)
              n141 = call-poly <vilib>:"Close.vi"("error in (no error)"=w217, "node"=w223) -> ("error out"=w219:errorcluster)  [unwired: 7 in]
            }
            "Array 4" <- w202
            n142 = call-poly <vilib>:"Close.vi"("error in (no error)"=w205, "node"=w208) -> ()  [unwired: 8 out]
          }
          frame Disabled {
            n143 = Open/Create/Replace File(file path (use dialog)=w302, access (0:read/write)=enum16{"read/write", "read-only", "write-only"}."read-only") -> (refnum out=w309:refnum<file>, error out=w308:errorcluster)  [unwired: 4 in, 1 out]
            n144 = Read from Text File(file (use dialog)=w309, error in=w308) -> (refnum out=w307:refnum<file>, text=w305:string, error out=w306:errorcluster)  [unwired: 2 in, 1 out]
            n145 = Close File(refnum=w307, error in=w306) -> (path=w303:path)  [unwired: 1 out]
            n146 = while {
              shift-right: [w318] -> _
              shift-left: w305 -> [w322]
              tunnel: [w317] -> w304 mode=indexing if=w313
              tunnel: w303 -> [w312]
              stop <- w319 stop-if-true
              n147 = Match Pattern(string=w322, regular expression="<Item") -> (after substring=w311:string, offset past match=w320:i32)  [unwired: 1 in, 2 out]
              n148 = Match Pattern(string=w311, regular expression="Type=\"VI\"") -> (match substring=w314:string, after substring=w315:string)  [unwired: 1 in, 2 out]
              n149 = case shown="\"Type=\\\"VI\\\"\"" w314 {
                tunnel: [w323 w353] -> w318
                tunnel: [_ w350] -> w317
                tunnel: w315 -> [_ w352]
                tunnel: [FALSE w325] -> w313
                tunnel: w312 -> [_ w351]
                tunnel: w311 -> [w323 _]
                frame Default {
                }
                frame "Type=\"VI\"" {
                  n150 = Path To String(path=path "") -> (string=w329:string)
                  n151 = Match Pattern(string=w352, regular expression="</Item>") -> (before substring=w346:string, after substring=w353:string)  [unwired: 1 in, 2 out]
                  n152 = Match Pattern(string=w352, regular expression="URL=\"[~\"]*\"") -> (match substring=w340:string)  [unwired: 1 in, 3 out]
                  n153 = Empty String/Path?(string/path=w329) -> (empty?=w331:bool)
                  n154 = Select(t="\\" ("search string"), s=w331, f=w329) -> (s? t:f=w333:string)
                  n155 = String Subset(string=w340, offset (0)=4) -> (substring=w339:string)  [unwired: 1 in]
                  n156 = Match Pattern(string=w346, regular expression="NI.ClassItem.IsStaticMethod" ("format string")) -> (after substring=w345:string)  [unwired: 1 in, 3 out]
                  n157 = Search and Replace String(replace all?=TRUE ("replace all? (F)"), input string=w339, search string="\"", replace string="") -> (result string=w334:string)  [unwired: 4 in, 3 out]
                  n158 = Search and Replace String(replace all?=TRUE ("replace all? (F)"), input string=w334, search string="/", replace string=w333) -> (result string=w335:string)  [unwired: 4 in, 3 out]
                  n159 = Match Pattern(string=w345, regular expression="</Property>") -> (before substring=w328:string)  [unwired: 1 in, 3 out]
                  n160 = Build Path(base path=w351, name or relative path=w335) -> (appended path=w350:path)
                  n161 = Match Pattern(string=w328, regular expression="true") -> (offset past match=w326:i32)  [unwired: 1 in, 3 out]
                  n162 = Greater Or Equal To 0?(x=w326) -> (x >= 0?=w325:bool)
                }
              }
              n163 = Less Than 0?(x=w320) -> (x < 0?=w319:bool)
            }
            "Array 3" <- w304
          }
          frame Disabled {
            n164 = call <vilib>:"Get LV Class Path.vi"("object"=refnum<class "Test Case Test Double.lvclass"> refnum ("Test Case Test Double.lvclass")) -> ("class path"=w362:path)  [unwired: 9 in, 1 out]
            n165 = Open/Create/Replace File(file path (use dialog)=w362, access (0:read/write)=enum16{"read/write", "read-only", "write-only"}."read-only") -> (refnum out=w360:refnum<file>, error out=w359:errorcluster)  [unwired: 4 in, 1 out]
            n166 = Read from Text File(file (use dialog)=w360, error in=w359) -> (refnum out=w358:refnum<file>, text=w356:string, error out=w357:errorcluster)  [unwired: 2 in, 1 out]
            n167 = Close File(refnum=w358, error in=w357) -> (path=w354:path)  [unwired: 1 out]
            n168 = while {
              shift-right: [w371] -> _
              shift-left: w356 -> [w375]
              tunnel: [w370] -> w355 mode=indexing if=w366
              tunnel: w354 -> [w365]
              stop <- w372 stop-if-true
              n169 = Match Pattern(string=w375, regular expression="<Item") -> (after substring=w364:string, offset past match=w373:i32)  [unwired: 1 in, 2 out]
              n170 = Match Pattern(string=w364, regular expression="Type=\"VI\"") -> (match substring=w367:string, after substring=w368:string)  [unwired: 1 in, 2 out]
              n171 = case shown="\"Type=\\\"VI\\\"\"" w367 {
                tunnel: [w376 w414] -> w371
                tunnel: [_ w411] -> w370
                tunnel: w368 -> [_ w413]
                tunnel: [FALSE w379] -> w366
                tunnel: w365 -> [_ w412]
                tunnel: w364 -> [w376 _]
                frame Default {
                }
                frame "Type=\"VI\"" {
                  n172 = Match Pattern(string=w413, regular expression="URL=\"[~\"]*\"") -> (match substring=w402:string)  [unwired: 1 in, 3 out]
                  n173 = Path To String(path=path "") -> (string=w391:string)
                  n174 = Empty String/Path?(string/path=w391) -> (empty?=w393:bool)
                  n175 = String Subset(string=w402, offset (0)=4) -> (substring=w401:string)  [unwired: 1 in]
                  n176 = Select(t="\\" ("search string"), s=w393, f=w391) -> (s? t:f=w395:string)
                  n177 = Search and Replace String(replace all?=TRUE ("replace all? (F)"), input string=w401, search string="\"", replace string="") -> (result string=w396:string)  [unwired: 4 in, 3 out]
                  n178 = Search and Replace String(replace all?=TRUE ("replace all? (F)"), input string=w396, search string="/", replace string=w395) -> (result string=w397:string)  [unwired: 4 in, 3 out]
                  n179 = Build Path(base path=w412, name or relative path=w397) -> (appended path=w411:path)
                  n180 = Match Pattern(string=w413, regular expression="</Item>") -> (before substring=w383:string, after substring=w414:string)  [unwired: 1 in, 2 out]
                  n181 = Match Pattern(string=w383, regular expression="NI.ClassItem.MethodScope" ("format string")) -> (after substring=w386:string)  [unwired: 1 in, 3 out]
                  n182 = Match Pattern(string=w383, regular expression="NI.ClassItem.IsStaticMethod" ("format string")) -> (after substring=w407:string)  [unwired: 1 in, 3 out]
                  n183 = Match Pattern(string=w386, regular expression="</Property>") -> (before substring=w380:string)  [unwired: 1 in, 3 out]
                  n184 = Match Pattern(string=w407, regular expression="</Property>") -> (before substring=w390:string)  [unwired: 1 in, 3 out]
                  n185 = Match Pattern(string=w380, regular expression="1") -> (offset past match=w382:i32)  [unwired: 1 in, 3 out]
                  n186 = Match Pattern(string=w390, regular expression="true") -> (offset past match=w388:i32)  [unwired: 1 in, 3 out]
                  n187 = Greater Or Equal To 0?(x=w382) -> (x >= 0?=w378:bool)
                  n188 = Greater Or Equal To 0?(x=w388) -> (x >= 0?=w387:bool)
                  n189 = And(x=w387, y=w378) -> (x .and. y?=w379:bool)
                }
              }
              n190 = Less Than 0?(x=w373) -> (x < 0?=w372:bool)
            }
            "Array 5" <- w355
          }
          frame Disabled {
            n191 = invoke class="App" method="LVClass.Open"("Path"=w415) -> ("LVClass.Open"=w418:refnum<vi>)  [unwired: 3 in, 3 out]
            n192 = property class="LVClassLibrary"(reference=w418) -> ("Static Member VIs"=w417:refnum<vi>[])  [unwired: 1 in, 2 out]
            n193 = for {
              tunnel: [w419] -> w416 mode=indexing if=w432
              tunnel: w417 -> [w421] mode=indexing
              n194 = property class="VI"(reference=w421) -> ("Name"=w420:string, "Path"=w419:path)  [unwired: 1 in, 2 out]
              n195 = To Lower Case(string=w420) -> (all lower case string=w423:string)
              n196 = Match Pattern(string=w423, regular expression="lvclass:") -> (after substring=w429:string)  [unwired: 1 in, 3 out]
              n197 = Match Pattern(string=w423, regular expression=".vit$") -> (offset past match=w434:i32)  [unwired: 1 in, 3 out]
              n198 = Match Pattern(string=w429, regular expression="^_*test") -> (offset past match=w431:i32)  [unwired: 1 in, 3 out]
              n199 = Match Pattern(string=w429, regular expression="^_*verify") -> (offset past match=w426:i32)  [unwired: 1 in, 3 out]
              n200 = Less Than 0?(x=w434) -> (x < 0?=w433:bool)
              n201 = Greater Or Equal To 0?(x=w431) -> (x >= 0?=w424:bool)
              n202 = Greater Or Equal To 0?(x=w426) -> (x >= 0?=w425:bool)
              n203 = Or(x=w424, y=w425) -> (x .or. y?=w422:bool)
              n204 = Compound Arithmetic op=AND(w422, w433) -> (w432:bool)
            }
          }
        }
        "Numeric" <- w14
      }
    }
    frame #2 {
      n205 = Tick Count (ms)() -> (millisecond timer value=w437:u32)
    }
  }
  n206 = Subtract(x=w8, y=w5) -> (x-y=→"x-y":u32)
